vi "Advanced Single Point Benchmark.vi"() -> ()   [LabVIEW 2011]
panel:
  in  "Configuration:Measurement Options:DC Noise Rejection":i32(ring)=2 items=["Auto"=-1, "Normal"=0, "Second_Order"=1, "High_Order"=2]
  in  "Configuration:Advanced:Settle Time":dbl=0.001
  in  "Configuration:Advanced:Aperture Time":dbl=0.1
  in  "Configuration:Advanced:Aperture Time Units":i32(ring) items=["NIDMM_VAL_SECONDS", "NIDMM_VAL_POWER_LINE_CYCLES"]
  in  "Configuration:Function":i32(ring)=1 items=["NIDMM_VAL_DC_VOLTS"=1, "NIDMM_VAL_AC_VOLTS"=2, "NIDMM_VAL_DC_CURRENT"=3, "NIDMM_VAL_AC_CURRENT"=4, "NIDMM_VAL_2_WIRE_RES"=5, "NIDMM_VAL_4_WIRE_RES"=101, "NIDMM_VAL_FREQ"=104, "NIDMM_VAL_PERIOD"=105, "NIDMM_VAL_AC_VOLTS_DC_COUPLED"=1001, "NIDMM_VAL_DIODE"=1002, "NIDMM_VAL_CAPACITANCE"=1005, "NIDMM_VAL_INDUCTANCE"=1006, "NIDMM_VAL_WAVEFORM_VOLTAGE"=1003, "NIDMM_VAL_WAVEFORM_CURRENT"=1004]
  in  "Configuration:Range":dbl=10.0
  in  "Configuration:Measurement Options:ADC Calibration":i32(ring)=1 items=["Auto"=-1, "Off"=0, "On"=1]
  in  "Configuration:Measurement Options:Auto Zero":i32(ring)=1 items=["Auto"=-1, "Off"=0, "On"=1, "Once"=2]
  out "Measurement Period (seconds)":dbl format="%.4f"
  in  "Instrument Descriptor":refnum<k15>="DMM"
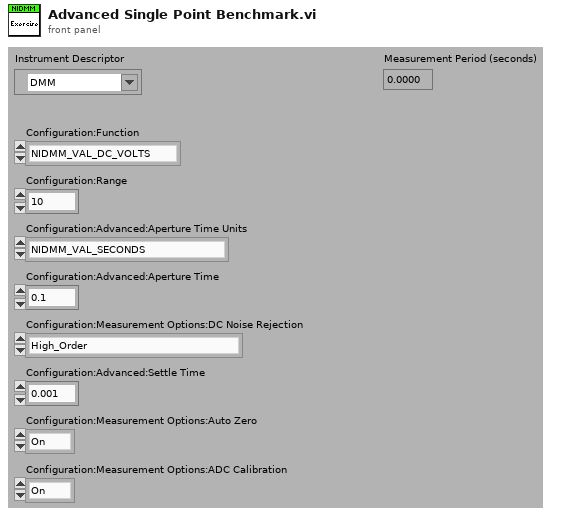
[diagram p1: front panel]
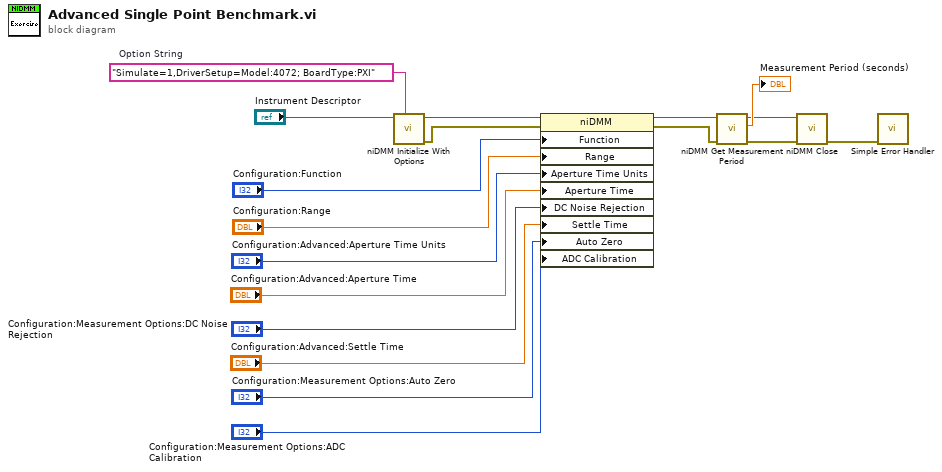
[diagram p0: block diagram]
diagram:
  w13 = "Simulate=1,DriverSetup=Model:4072; BoardType:PXI"  # Option String
  n1 = call <instrlib>:"niDMM Initialize With Options.vi"("Option String"=w13, "Instrument Descriptor"="Instrument Descriptor") -> ("error out"=w1:errorcluster, "instrument handle out"=w12:refnum<k15>)  [unwired: 8 in]
  n2 = property class="niDMM"(reference=w12, error in=w1, "Function"="Configuration:Function", "Range"="Configuration:Range", "Aperture Time Units"="Configuration:Advanced:Aperture Time Units", "Aperture Time"="Configuration:Advanced:Aperture Time", "DC Noise Rejection"="Configuration:Measurement Options:DC Noise Rejection", "Settle Time"="Configuration:Advanced:Settle Time", "Auto Zero"="Configuration:Measurement Options:Auto Zero", "ADC Calibration"="Configuration:Measurement Options:ADC Calibration") -> (reference out=w3:refnum<k15>, error out=w2:errorcluster)
  n3 = call <instrlib>:"niDMM Get Measurement Period.vi"("error in (no error)"=w2, "instrument handle"=w3) -> ("error out"=w16:errorcluster, "Measurement Period (seconds)"=→"Measurement Period (seconds)":dbl, "instrument handle out"=w15:refnum<k15>)  [unwired: 7 in]
  n4 = call <instrlib>:"niDMM Close.vi"("error in (no error)"=w16, "instrument handle"=w15) -> ("error out"=w14:errorcluster)  [unwired: 9 in]
  n5 = call <vilib>:"Simple Error Handler.vi"("error in (no error)"=w14) -> ()  [unwired: 4 in, 5 out]
